vi "TestTransforms.vi"(8 "error in (no error)":errorcluster) -> (0 "error out":errorcluster)   [LabVIEW 2019]
uses:
  Transform/Transform.lvclass
  <vilib>/Analysis/Matrix/Datatypes/RealMatrix.ctl
  Transform.Matrix/Transform.Matrix.lvclass
  C:/Users/Albro/Documents/GitHub/AFM-Lithography/lvsrc/Classes/Parse/Transform/Transform.lvclass
  Transform.Translate/Transform.Translate.lvclass
  Transform.Rotate/Transform.Rotate.lvclass
  Transform.Skew/Transform.Skew.lvclass
  Transform/Transform.lvclass/Transform.ctl
  <vilib>/addons/_JKI Toolkits/Caraya/classes/Assert/Assert Equal Value_Variant.vi
  <vilib>/Analysis/Matrix/Numeric/Conversions/Matrix To Array - RM.vi
  <vilib>/addons/_JKI Toolkits/Caraya/classes/Test/Test.lvclass
  <vilib>/addons/_JKI Toolkits/Caraya/classes/Assert/Assert.lvclass
  <vilib>/Analysis/Matrix/NI_Matrix.lvlib
panel:
  # "1"
  # "1"
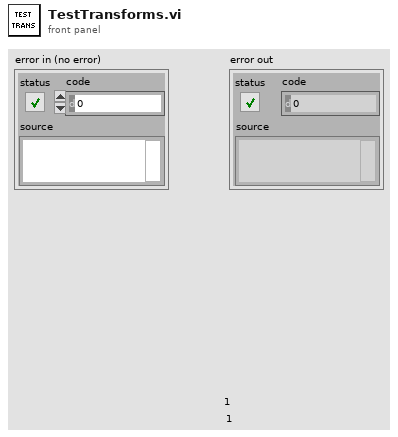
[diagram p1: front panel]
types:
  T1 = typedef "NI_Matrix.lvlib/RealMatrix.ctl" = dbl[][]
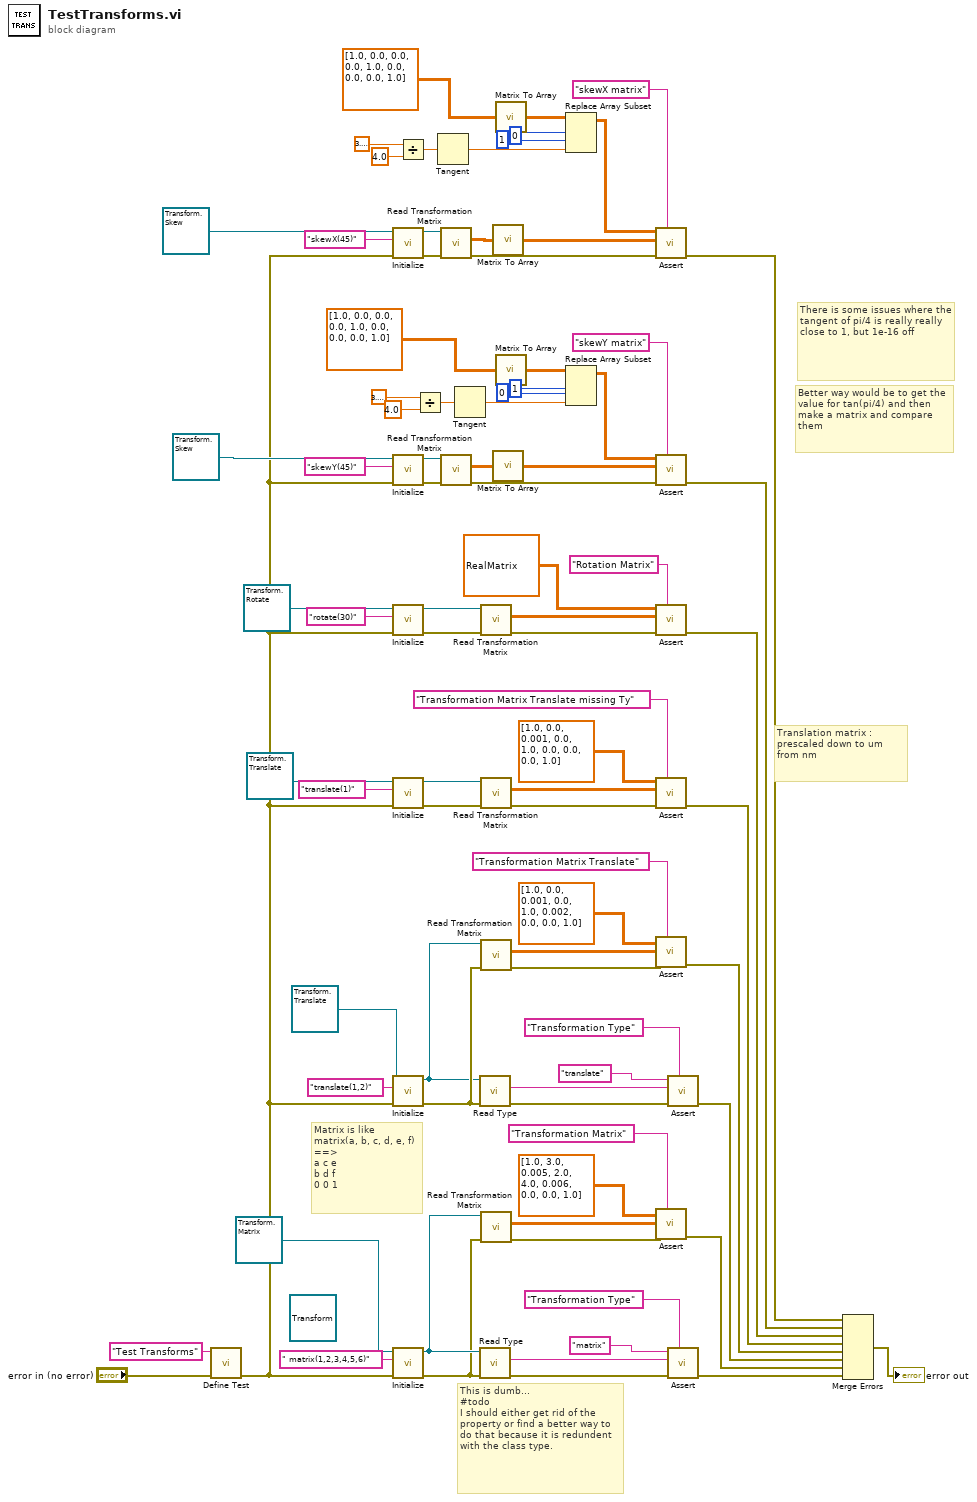
[diagram p0: block diagram]
diagram:
  (unwired) refnum<class "Transform.lvclass"> refnum ("Transform in")
  # "Translation matrix : prescaled down to um from nm"
  # "Better way would be to get the value for tan(pi/4) and then make a matrix and compare them"
  # "Matrix is like \nmatrix(a, b, c, d, e, f)\n==>\na c e\nb d f\n0 0 1"
  # "There is some issues where the tangent of pi/4 is really really close to 1, but 1e-16 off"
  # "This is dumb...\n#todo\nI should either get rid of the property or find a better way to do that because it is redundent with the class type."
  n1 = call <vilib>:"Define Test.vi"("error in (no error)"="error in (no error)", "Label (VI Title)"="Test Transforms") -> ("error out"=w19:errorcluster)  [unwired: 8 in, 1 out]
  n2 = call-dynamic "Initialize.vi"("error in (no error)"=w19, "Transform"="skewX(45)", "Transform in"=refnum<class "Transform.Skew.lvclass"> refnum ("Transform.Skew in")) -> ("error out"=w26:errorcluster, "Transform out"=w25:refnum<class "Transform.Skew.lvclass">)  [unwired: 7 in]
  n3 = call-dynamic "Initialize.vi"("error in (no error)"=w19, "Transform"="skewY(45)", "Transform in"=refnum<class "Transform.Skew.lvclass"> refnum ("Transform.Skew in")) -> ("error out"=w36:errorcluster, "Transform out"=w37:refnum<class "Transform.Skew.lvclass">)  [unwired: 7 in]
  n4 = call-dynamic "Initialize.vi"("error in (no error)"=w19, "Transform"="rotate(30)", "Transform in"=refnum<class "Transform.Rotate.lvclass"> refnum ("Transform.Rotate.lvclass")) -> ("error out"=w49:errorcluster, "Transform out"=w48:refnum<class "Transform.Rotate.lvclass">)  [unwired: 7 in]
  n5 = call-dynamic "Initialize.vi"("error in (no error)"=w19, "Transform"="translate(1)", "Transform in"=refnum<class "Transform.Translate.lvclass"> refnum ("Transform.Translate.lvclass")) -> ("error out"=w53:errorcluster, "Transform out"=w54:refnum<class "Transform.Translate.lvclass">)  [unwired: 7 in]
  n6 = call-dynamic "Initialize.vi"("error in (no error)"=w19, "Transform"="translate(1,2)", "Transform in"=refnum<class "Transform.Translate.lvclass"> refnum ("Transform.Translate.lvclass")) -> ("error out"=w65:errorcluster, "Transform out"=w64:refnum<class "Transform.Translate.lvclass">)  [unwired: 7 in]
  n7 = call-dynamic "Initialize.vi"("error in (no error)"=w19, "Transform"=" matrix(1,2,3,4,5,6)", "Transform in"=refnum<class "Transform.Matrix.lvclass"> refnum ("Transform.Matrix in")) -> ("error out"=w77:errorcluster, "Transform out"=w78:refnum<class "Transform.Matrix.lvclass">)  [unwired: 7 in]
  n8 = Divide(x=3.141592653589793, y=4.0) -> (x/y=w10:dbl)
  n9 = Divide(x=3.141592653589793, y=4.0) -> (x/y=w15:dbl)
  n10 = Tangent(1:w10) -> (0:w9:dbl)
  n11 = call "Read Transformation Matrix.vi"("error in (no error)"=w26, "Transform in"=w25) -> ("error out"=w23:errorcluster, "Real Matrix"=w20:T1)  [unwired: 7 in, 1 out]
  n12 = call "Read Transformation Matrix.vi"("error in (no error)"=w36, "Transform in"=w37) -> ("error out"=w39:errorcluster, "Real Matrix"=w42:T1)  [unwired: 7 in, 1 out]
  n13 = Tangent(1:w15) -> (0:w14:dbl)
  n14 = call "Read Type.vi"("error in (no error)"=w65, "Transform in"=w64) -> ("error out"=w60:errorcluster, "Type"=w61:string)  [unwired: 7 in, 1 out]
  n15 = call "Read Type.vi"("error in (no error)"=w77, "Transform in"=w78) -> ("error out"=w82:errorcluster, "Type"=w81:string)  [unwired: 7 in, 1 out]
  n16 = call "Read Transformation Matrix.vi"("error in (no error)"=w49, "Transform in"=w48) -> ("error out"=w46:errorcluster, "Real Matrix"=w44:T1)  [unwired: 7 in, 1 out]
  n17 = call "Read Transformation Matrix.vi"("error in (no error)"=w53, "Transform in"=w54) -> ("error out"=w58:errorcluster, "Real Matrix"=w57:T1)  [unwired: 7 in, 1 out]
  n18 = call "Read Transformation Matrix.vi"("error in (no error)"=w65, "Transform in"=w64) -> ("error out"=w66:errorcluster, "Real Matrix"=w67:T1)  [unwired: 7 in, 1 out]
  n19 = call "Read Transformation Matrix.vi"("error in (no error)"=w77, "Transform in"=w78) -> ("error out"=w76:errorcluster, "Real Matrix"=w75:T1)  [unwired: 7 in, 1 out]
  n20 = call-poly <vilib>:"Matrix To Array.vi"("Real Matrix"=w20) -> ("Real 2D Array"=w8:dbl[][])
  n21 = call-poly <vilib>:"Matrix To Array.vi"("Real Matrix"=w42) -> ("Real 2D Array"=w13:dbl[][])
  n22 = call-poly <vilib>:"Matrix To Array.vi"("Real Matrix"=T1 [[1.0, 0.0, 0.0], [0.0, 1.0, 0.0], [0.0, 0.0, 1.0]] ("appended array")) -> ("Real 2D Array"=w21:dbl[][])
  n23 = call-poly <vilib>:"Matrix To Array.vi"("Real Matrix"=T1 [[1.0, 0.0, 0.0], [0.0, 1.0, 0.0], [0.0, 0.0, 1.0]] ("appended array")) -> ("Real 2D Array"=w41:dbl[][])
  n24 = Replace Array Subset(array=w21, new element=w9, index (row)=0 ("length"), index (col)=1 ("index (row)")) -> (w29:dbl[][])
  n25 = Replace Array Subset(array=w41, new element=w14, index (row)=1 ("length"), index (col)=0 ("index (row)")) -> (w33:dbl[][])
  n26 = call-poly <vilib>:"Assert.vi"("Label"="skewX matrix", "error in (no error)"=w23, "Y"=w8, "X"=w29) -> ("error out"=w5:errorcluster)  [unwired: 6 in, 1 out]
  n27 = call-poly <vilib>:"Assert.vi"("Label"="skewY matrix", "error in (no error)"=w39, "Y"=w13, "X"=w33) -> ("error out"=w6:errorcluster)  [unwired: 6 in, 1 out]
  n28 = call-poly <vilib>:"Assert.vi"("Label"="Rotation Matrix", "error in (no error)"=w46, "Y"=w44, "X"=T1 [[0.8660254037844387, -0.49999999999999994, 0.0], [0.49999999999999994, 0.8660254037844387, 0.0], [0.0, 0.0, 1.0]] ("appended array")) -> ("error out"=w7:errorcluster)  [unwired: 6 in, 1 out]
  n29 = call-poly <vilib>:"Assert.vi"("Label"="Transformation Matrix Translate missing Ty", "error in (no error)"=w58, "Y"=w57, "X"=T1 [[1.0, 0.0, 0.001], [0.0, 1.0, 0.0], [0.0, 0.0, 1.0]] ("appended array")) -> ("error out"=w4:errorcluster)  [unwired: 6 in, 1 out]
  n30 = call-poly <vilib>:"Assert.vi"("Label"="Transformation Matrix Translate", "error in (no error)"=w66, "Y"=w67, "X"=T1 [[1.0, 0.0, 0.001], [0.0, 1.0, 0.002], [0.0, 0.0, 1.0]] ("appended array")) -> ("error out"=w3:errorcluster)  [unwired: 6 in, 1 out]
  n31 = call-poly <vilib>:"Assert.vi"("Label"="Transformation Matrix", "error in (no error)"=w76, "Y"=w75, "X"=T1 [[1.0, 3.0, 0.005], [2.0, 4.0, 0.006], [0.0, 0.0, 1.0]] ("appended array")) -> ("error out"=w1:errorcluster)  [unwired: 6 in, 1 out]
  n32 = call-poly <vilib>:"Assert.vi"("Label"="Transformation Type", "error in (no error)"=w60, "Y"=w61, "X"="translate" ("Type")) -> ("error out"=w2:errorcluster)  [unwired: 6 in, 1 out]
  n33 = call-poly <vilib>:"Assert.vi"("Label"="Transformation Type", "error in (no error)"=w82, "Y"=w81, "X"="matrix" ("Type")) -> ("error out"=w84:errorcluster)  [unwired: 6 in, 1 out]
  n34 = Merge Errors(w5, w6, w7, w4, w3, w2, w1, w84) -> (→"error out":errorcluster)
